vi "Write Enable.vi"(10 "Enable":bool=TRUE, 11 "DA in":refnum<class "DA.lvclass">) -> (3 "DA out":refnum<class "DA.lvclass">)   [LabVIEW 2019, in "DA.lvclass"]
uses:
  DA.lvclass
  DA.lvclass/DA.ctl
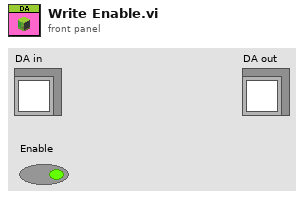
[diagram p1: front panel]
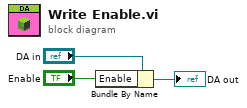
[diagram p0: block diagram]
diagram:
  n1 = Bundle By Name(cluster="DA in", "Enable"="Enable") -> (→"DA out":refnum<class "DA.lvclass">)
